vi "Trial Timestamp.vi"(8 "error in (no error)":errorcluster, 11 "TrialBasedExperiment in":refnum<class "TrialBasedExperiment.lvclass">) -> (0 "error out":errorcluster, 3 "TrialBasedExperiment out":refnum<class "TrialBasedExperiment.lvclass">)   [LabVIEW 2012, in "AcquisitionCoreObjects.lvlib" / "TrialBasedExperiment.lvclass"]
uses:
  TrialBasedExperiment.lvclass
  Acquisition/AcquistionObject/AcquistionObject.lvclass
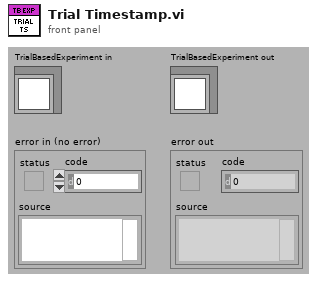
[diagram p1: front panel]
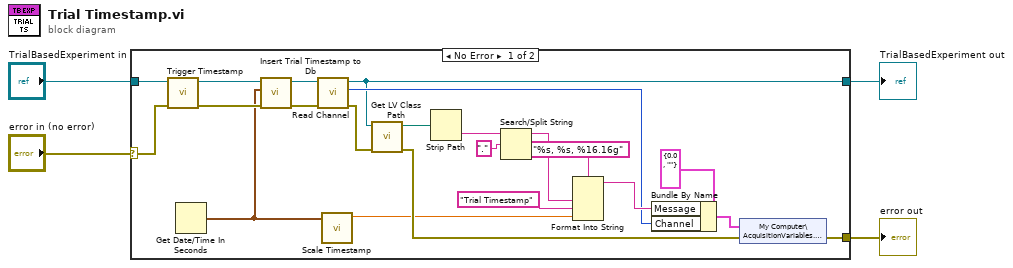
[diagram p0: block diagram]
diagram:
  n1 = case shown="No Error" "error in (no error)" {
    selector: "error in (no error)" -> [w26 w28]
    tunnel: [w13 w28] -> w3
    tunnel: [w12 w27] -> w1
    tunnel: "TrialBasedExperiment in" -> [w25 w27]
    frame No Error {
      n2 = call-dynamic "Trigger Timestamp.vi"("error in (no error)"=w26, "TrialBasedExperiment in"=w25) -> ("error out"=w8:errorcluster, "TrialBasedExperiment out"=w9:refnum<class "TrialBasedExperiment.lvclass">)  [unwired: 8 in]
      n3 = Get Date/Time In Seconds() -> (seconds since 1Jan1904=w5:timestamp)
      n4 = call-dynamic "Insert Trial Timestamp to Db.vi"("error in (no error)"=w8, "Timetsamp Time"=w5, "TrialBasedExperiment in"=w9) -> ("error out"=w7:errorcluster, "TrialBasedExperiment out"=w6:refnum<class "TrialBasedExperiment.lvclass">)  [unwired: 7 in]
      n5 = call-dynamic "Read Channel.vi"("error in (no error)"=w7, "AcquistionObject in"=w6) -> ("error out"=w14:errorcluster, "Channel"=w15:i16, "AcquistionObject out"=w12:refnum<class "TrialBasedExperiment.lvclass">)  [unwired: 7 in]
      n6 = call "Scale Timestamp.vi"("Time Stamp"=w5) -> ("Scaled timestamp"=w10:dbl)  [unwired: 10 in]
      n7 = call <vilib>:"Get LV Class Path.vi"("error in (no error)"=w14, "object"=w12) -> ("error out"=w16:errorcluster, "class path"=w20:path)  [unwired: 8 in]
      n8 = Strip Path(path=w20) -> (name=w18:string)  [unwired: 1 out]
      n9 = Search/Split String(string=w18, search string/char (-)=".") -> (substring before match=w17:string)  [unwired: 1 in, 2 out]
      n10 = Format Into String(format string="%s, %s, %16.16g", w17, "Trial Timestamp" ("input 2"), w10) -> (resulting string=w21:string)  [unwired: 2 in, 1 out]
      n11 = Bundle By Name(cluster=cluster{"Channel":dbl, "Message":string} {"Channel"=0.0, "Message"=""} ("Message"), "Message"=w21, "Channel"=w15) -> (w24:cluster{"Channel":dbl, "Message":string})
      n12 = shared-variable "My Computer\\AcquisitionVariables.lvlib\\Message"(w24, error in=w16) -> (error out=w13:errorcluster)
    }
    frame Error {
    }
  }
  "error out" <- w3
  "TrialBasedExperiment out" <- w1
